vi "Write Serial Configs.vi"(8 "error in (no error)":errorcluster, 10 "Item Ref in":T2 format="%.0x", 11 "Refnum in":T1) -> (0 "error out":errorcluster, 2 "Item Ref out":T2 format="%.0x", 3 "Refnum out":T1)   [LabVIEW 2021, in "Modbus Master System Explorer.lvlib"]
uses:
  Modbus Master System Explorer.lvlib
  <vilib>/Utility/config.llb/Config Data RefNum.ctl
  <vilib>/NI VeriStand/Custom Device API/Custom Device Item Ref.ctl
  <vilib>/Utility/config.llb/Write Key (String).vi
  <vilib>/Utility/config.llb/Write Key (U32).vi
  <vilib>/Utility/config.llb/NI_LVConfig.lvlib
  <vilib>/NI VeriStand/Custom Device API/Custom Device API.lvlib
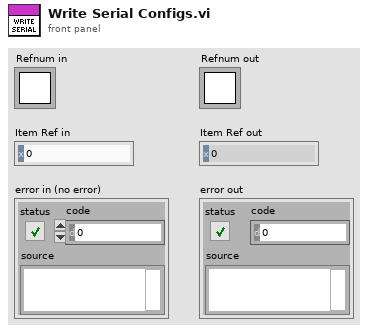
[diagram p1: front panel]
types:
  T1 = typedef "NI_LVConfig.lvlib/Config Data RefNum.ctl" = refnum<k1>
  T2 = typedef "Custom Device API.lvlib/Custom Device Item Ref.ctl" = u64
  T3 = typedef "Modbus Master Shared.lvlib/Parity.ctl" = u16
  T4 = typedef "Modbus Master Shared.lvlib/Serial Type.ctl" = enum16{"RTU", "ASCII"}
  T5 = typedef "Modbus Master Shared.lvlib/Flow Control.ctl" = u16
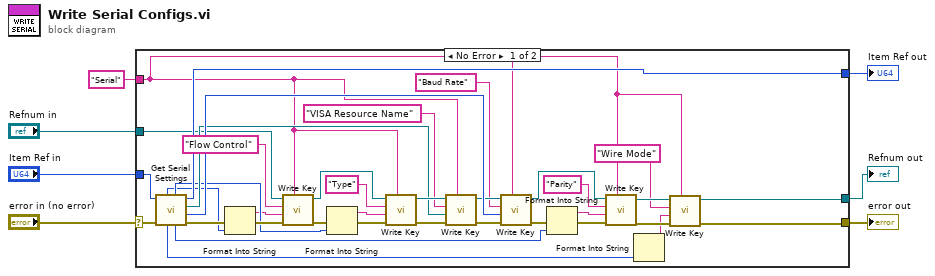
[diagram p0: block diagram]
diagram:
  n1 = case shown="No Error" "error in (no error)" {
    selector: "error in (no error)" -> [w17 w45]
    tunnel: [w13 w46] -> w7
    tunnel: [w12 w45] -> w6
    tunnel: [w43 w47] -> w5
    tunnel: "Serial" ("section") -> [w11 _]
    tunnel: "Item Ref in" -> [w18 w47]
    tunnel: "Refnum in" -> [w16 w46]
    frame No Error {
      n2 = call "Get Serial Settings.vi"("error in (no error)"=w17, "Item Ref in"=w18) -> ("error out"=w25:errorcluster, "baud rate"=w36:u32, "VISA resource name"=w30:refnum<visa-resource-name>, "Item Ref out"=w43:T2, "parity (even)"=w39:T3, "serial type"=w23:T4, "Wire Mode"=w9:i32, "flow control (none)"=w20:T5)  [unwired: 2 in]
      n3 = Format Into String(error in=w25, w20) -> (resulting string=w21:string, error out=w26:errorcluster)  [unwired: 2 in]
      n4 = call-poly <vilib>:"Write Key.vi"("section"=w11, "error in (no error)"=w26, "value"=w21, "key"="Flow Control", "refnum"=w16) -> ("error out"=w27:errorcluster, "refnum out"=w33:T1)  [unwired: 4 in, 1 out]
      n5 = Format Into String(error in=w27, w23) -> (resulting string=w24:string, error out=w28:errorcluster)  [unwired: 2 in]
      n6 = call-poly <vilib>:"Write Key.vi"("section"=w11, "error in (no error)"=w28, "value"=w24, "key"="Type", "refnum"=w33) -> ("error out"=w31:errorcluster, "refnum out"=w32:T1)  [unwired: 4 in, 1 out]
      n7 = call-poly <vilib>:"Write Key.vi"("section"=w11, "error in (no error)"=w31, "value"=w30, "key"="VISA Resource Name", "refnum"=w32) -> ("error out"=w37:errorcluster, "refnum out"=w35:T1)  [unwired: 4 in, 1 out]
      n8 = call-poly <vilib>:"Write Key.vi"("section"=w11, "error in (no error)"=w37, "value"=w36, "key"="Baud Rate", "refnum"=w35) -> ("error out"=w41:errorcluster, "refnum out"=w44:T1)  [unwired: 4 in, 1 out]
      n9 = Format Into String(error in=w41, w39) -> (resulting string=w40:string, error out=w42:errorcluster)  [unwired: 2 in]
      n10 = call-poly <vilib>:"Write Key.vi"("section"=w11, "error in (no error)"=w42, "value"=w40, "key"="Parity", "refnum"=w44) -> ("error out"=w14:errorcluster, "refnum out"=w15:T1)  [unwired: 4 in, 1 out]
      n11 = Format Into String(w9) -> (resulting string=w8:string)  [unwired: 3 in, 1 out]
      n12 = call-poly <vilib>:"Write Key.vi"("section"=w11, "error in (no error)"=w14, "value"=w8, "key"="Wire Mode", "refnum"=w15) -> ("error out"=w12:errorcluster, "refnum out"=w13:T1)  [unwired: 4 in, 1 out]
    }
    frame Error {
    }
  }
  "Refnum out" <- w7
  "error out" <- w6
  "Item Ref out" <- w5
